vi "Main Rect3D.vi"() -> ()   [LabVIEW 2017]
uses:
  3DButton Handler/3DButton Handler.lvclass
  C:/Program Files (x86)/National Instruments/LabVIEW 2017/vi.lib/LIEF/Image Editor Handler/Image Editor Handler.lvclass
  Rectangle3D/Rectangle3D.lvclass
  C:/Program Files (x86)/National Instruments/LabVIEW 2017/vi.lib/LIEF/Forms/Shape/Shape.lvclass
  <vilib>/LIEF/Image Editor Handler/Image Editor Handler.lvclass
  <vilib>/LIEF/Forms/Shape/Shape.lvclass
panel:
  in  "2D Picture":picture
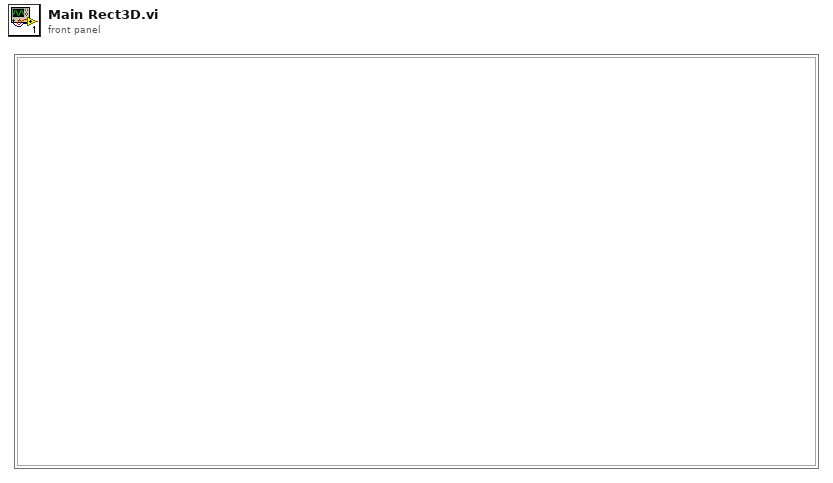
[diagram p1: front panel]
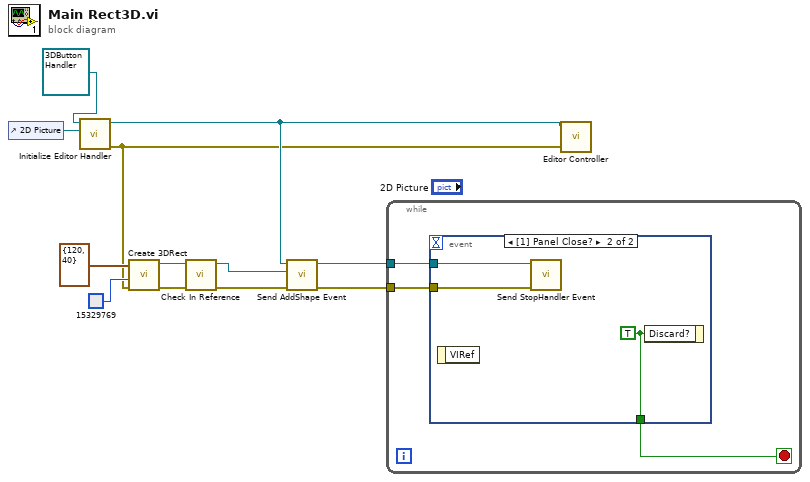
[diagram p0: block diagram]
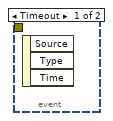
[diagram p2: hidden frame]
diagram:
  n1 = control-ref of="2D Picture"() -> (w12:refnum<vi>)
  n2 = call <vilib>:"Initialize Editor Handler.vi"("PictureRef"=w12, "Editor Handler in"=refnum<class "3DButton Handler.lvclass"> refnum ("3DButton Handler.lvclass")) -> ("error out"=w8:errorcluster, "Editor Handler out"=w9:refnum<class "3DButton Handler.lvclass">)  [unwired: 8 in]
  n3 = call "Create 3DRect.vi"("error in (no error)"=w8, "Color"=u32 15329769, "Size"=cluster{"Width":i32, "Height":i32} {"Width"=120, "Height"=40}) -> ("error out"=w7:errorcluster, "Rectangle3D out"=w6:refnum<class "Rectangle3D.lvclass">)  [unwired: 7 in]
  n4 = call <vilib>:"Check In Reference.vi"("error in (no error)"=w7, "Shape in"=w6) -> ("error out"=w4:errorcluster, "Shape Reference"=w5:refnum<data-value>)  [unwired: 8 in]
  n5 = call <vilib>:"Send AddShape Event.vi"("error in (no error)"=w4, "New Shape Reference"=w5, "Editor Handler in"=w9) -> ("error out"=w3:errorcluster, "Editor Handler out"=w2:refnum<class "3DButton Handler.lvclass">)  [unwired: 7 in]
  n6 = while {
    tunnel: w2 -> [w15]
    tunnel: w3 -> [w13]
    stop <- w14 stop-if-true
    n7 = event shown="[1] Panel Close?" {
      selector: _ -> [_ _]
      dyn-events: _ -> [_ _]
      timeout: _ -> [_ _]
      tunnel: w15 -> [_ w18]
      tunnel: [_ w17] -> w14
      tunnel: w13 -> [_ w16]
      event Timeout {
        n8 = event-data() -> ()  [unwired: 1 in, 3 out]
      }
      event Panel Close? {
        w17 = TRUE ("Discard?")
        n9 = event-data() -> ()  [unwired: 1 in, 1 out]
        n10 = call <vilib>:"Send StopHandler Event.vi"("error in (no error)"=w16, "Editor Handler in"=w18) -> ()  [unwired: 8 in, 2 out]
        n11 = event-data("Discard?"=w17) -> ()  [unwired: 1 in, 1 out]
      }
    }
  }
  n12 = call <vilib>:"Editor Controller.vi"("error in (no error)"=w8, "Editor Handler in"=w9) -> ()  [unwired: 8 in, 2 out]
